vi "HEWH Variable Scan Rate.vi"(6 "Purge Time (Seconds)":T1=180.0 format="%.2f", 7 "State":T2, 8 "error in (no error)":errorcluster, 10 "Elapsed Time (sec) in":dbl, 11 "Digital in":refnum<vi>) -> (0 "error out":errorcluster)   [LabVIEW 2019]
uses:
  Type Definitions/HEWH Purge Draw.ctl
  Utility/Custom Pallet Controls/Custom Pallet DBL.ctl
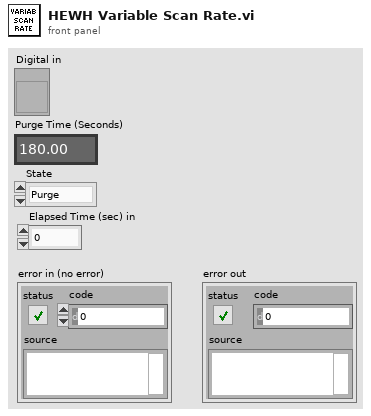
[diagram p1: front panel]
types:
  T1 = typedef "Custom Pallet DBL.ctl" = dbl
  T2 = typedef "HEWH Purge Draw.ctl" = enum16{"Purge", "Draw"}
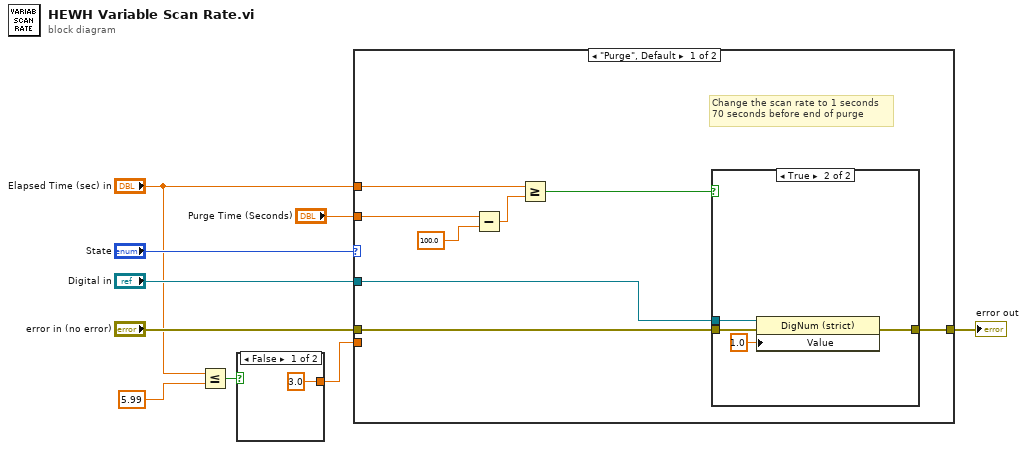
[diagram p0: block diagram]
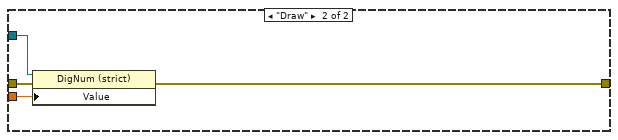
[diagram p3: hidden frame]
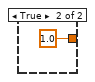
[diagram p4: hidden frame]
diagram:
  n1 = Less Or Equal?(x="Elapsed Time (sec) in", y=5.99) -> (x <= y?=w5:bool)
  n2 = case shown="False" w5 {
    tunnel: [3.0 ("y") 1.0 ("y")] -> w4
    frame False {
    }
    frame True {
    }
  }
  n3 = case shown="\"Purge\", Default" "State" {
    tunnel: "Digital in" -> [w12 w28]
    tunnel: [w13 w27] -> w8
    tunnel: "error in (no error)" -> [w14 w26]
    tunnel: w4 -> [_ w25]
    tunnel: "Elapsed Time (sec) in" -> [w19 _]
    tunnel: "Purge Time (Seconds)" -> [w18 _]
    frame "Purge", Default {
      # "Change the scan rate to 1 seconds\n70 seconds before end of purge"
      n4 = Subtract(x=w18, y=T1 100.0) -> (x-y=w16:T1)
      n5 = Greater Or Equal?(x=w19, y=w16) -> (x >= y?=w15:bool)
      n6 = case shown="True" w15 {
        tunnel: w14 -> [w20 w24]
        tunnel: [w20 w23] -> w13
        tunnel: w12 -> [_ w22]
        frame False {
        }
        frame True {
          n7 = property class="DigNum (strict)"(reference=w22, error in=w24, "Value"=T1 1.0) -> (error out=w23:errorcluster)  [unwired: 1 out]
        }
      }
    }
    frame "Draw" {
      n8 = property class="DigNum (strict)"(reference=w28, error in=w26, "Value"=w25) -> (error out=w27:errorcluster)  [unwired: 1 out]
    }
  }
  "error out" <- w8
